vi "Read Active.vi"(8 "error in":errorcluster, 11 "Alicat in":refnum<class "Alicat.lvclass">) -> (0 "error out":errorcluster, 2 "Active?":bool, 3 "Alicat out":refnum<class "Alicat.lvclass">)   [LabVIEW 2014, in "Alicat.lvlib" / "Alicat.lvclass"]
uses:
  Alicat.lvclass
  Alicat.lvclass/Alicat.ctl
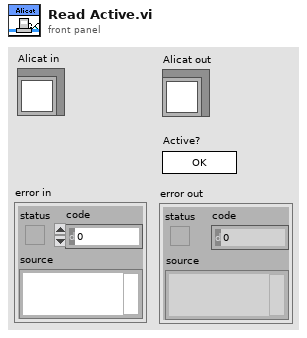
[diagram p1: front panel]
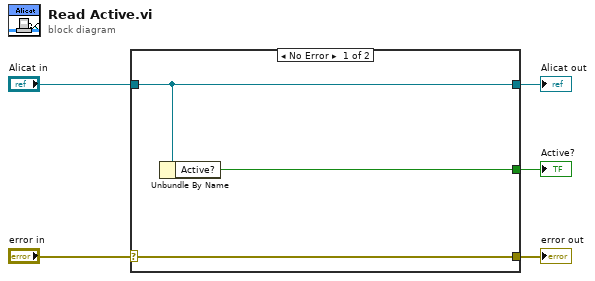
[diagram p0: block diagram]
diagram:
  n1 = case shown="No Error" "error in" {
    selector: "error in" -> [w8 w9]
    tunnel: [w8 w9] -> w4
    tunnel: [w7 w10] -> w2
    tunnel: "Alicat in" -> [w7 w10]
    tunnel: [w6 _] -> w1
    frame No Error {
      n2 = Unbundle By Name(w7) -> ("Active?"=w6:bool)
    }
    frame Error {
    }
  }
  "error out" <- w4
  "Alicat out" <- w2
  "Active?" <- w1
